vi "CRYInsert Waveform.vi"(8 "sOptionUpdate":string, 9 "sOption":string, 10 "Index":i32[](array[numeric]), 11 "Waveform":T1 {"Y dB ref" format="%.1f"; "Y axis" items=["Log", "Lin"]; "Y data" items=["dB", "Lin"]; "X data" items=["dB", "Lin"]}) -> (2 "Inserted Index":i32[](array[numeric]), 3 "Inserted Name Out":string[](array[string]))   [LabVIEW 2013]
uses:
  CRYSystem/Typedef Control/CRYWaveform Cluster Array.ctl
  CRYSystem/Typedef Control/CRYWaveform Cluster.ctl
  Global/CRYCurve Library Global.vi
  CRYSystem/Task Sequence/CRYProject Run Control Global.vi
  Global/CRYCurves Array Global.vi
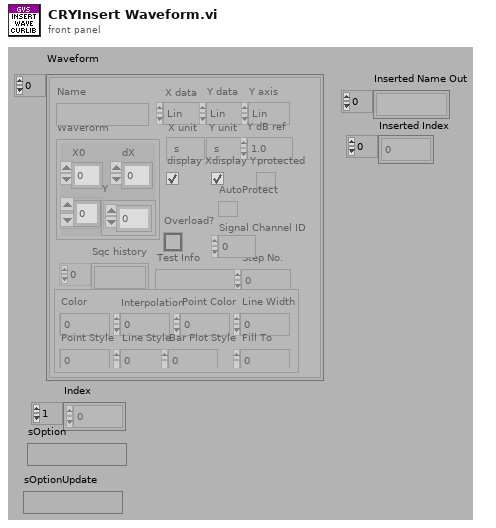
[diagram p1: front panel]
types:
  T1 = typedef "CRYWaveform Cluster Array.ctl" = T2[]
  T2 = typedef "CRYWaveform Cluster.ctl" = cluster{"Waveform":cluster{"X0":dbl, "dX":dbl, "Y":sgl[]}, "X data":u16, "Y data":u16, "Y axis":u16, "X unit":string, "Y unit":string, "Y dB ref":dbl, "display Y":bool, "display X":bool, "Overload?":bool, "Test Info":string, "Step No.":i32, "Name":string, "protected":bool, "Sqc history":string[], "Signal Channel ID":i32, "Plot Settings":cluster{"Color":u32, "Interpolation":u8, "Point Style":u8, "Line Style":u8, "Point Color":u32, "Line Width":u8, "Bar Plot Style":u8, "Fill To":i16}, "AutoProtect":bool}
  T3 = cluster{"Color":u32, "Interpolation":u8, "Point Style":u8, "Line Style":u8, "Point Color":u32, "Line Width":u8, "Bar Plot Style":u8, "Fill To":i16}
  T4 = cluster{"CurveOld":string[], "ValueOld":string[], "ResultOld":string[], "WFMOld":string[], "CurveNew":string[], "ValueNew":string[], "ResultNew":string[], "WFMNew":string[]}
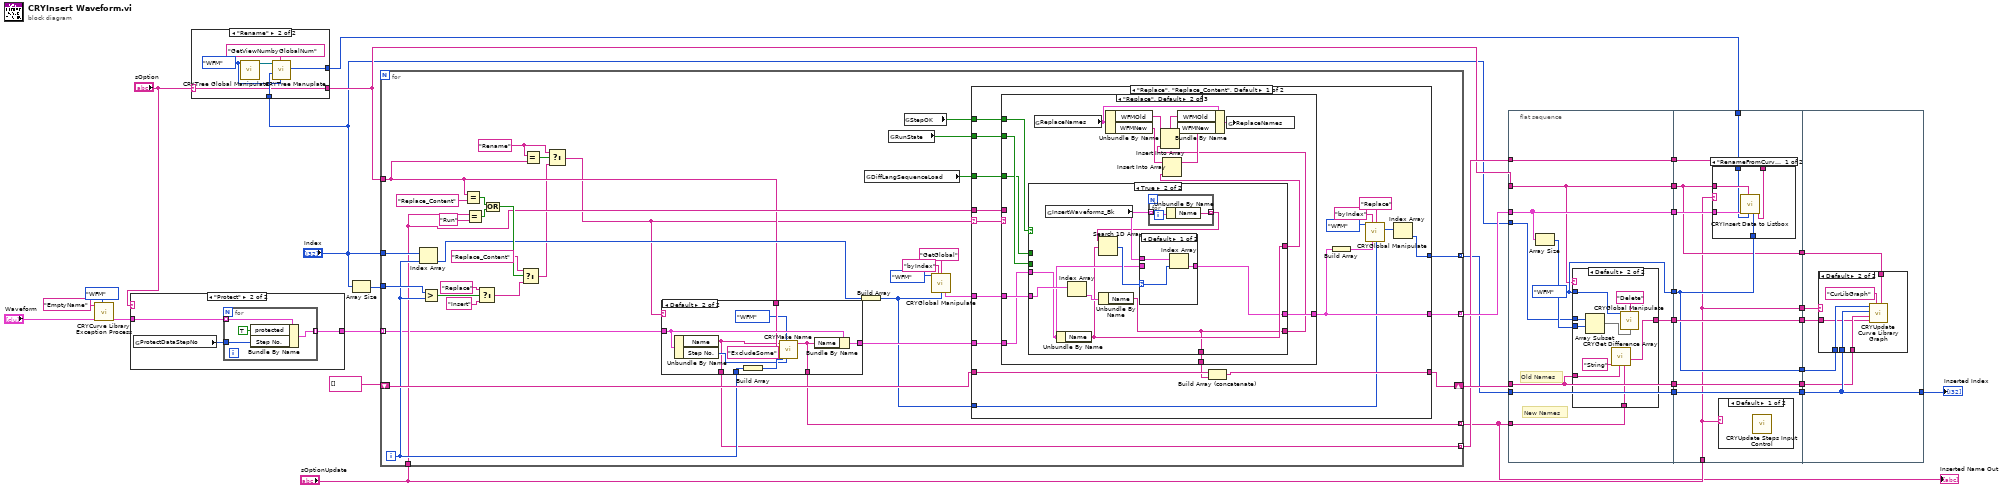
[diagram p0: block diagram]
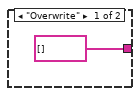
[diagram p4: hidden frame]
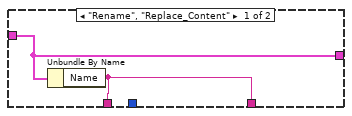
[diagram p8: hidden frame]
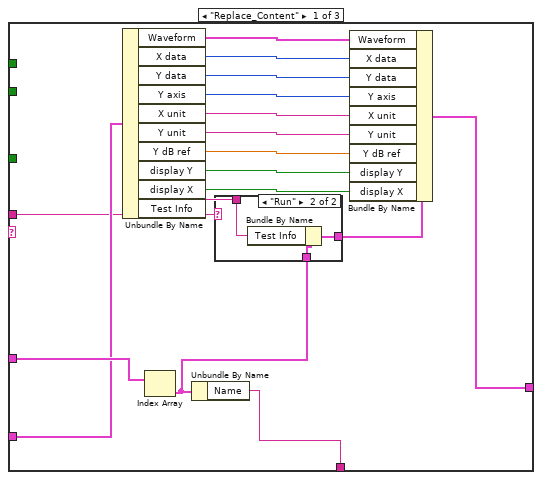
[diagram p9: hidden frame]
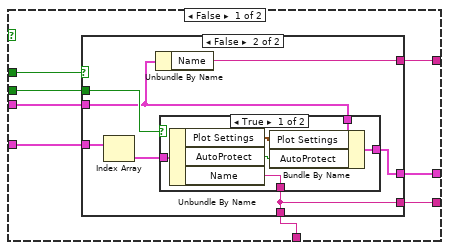
[diagram p11: hidden frame]
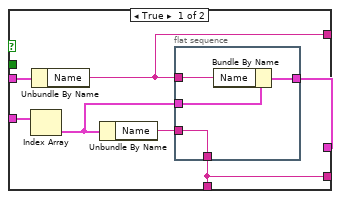
[diagram p12: hidden frame]
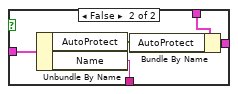
[diagram p13: hidden frame]
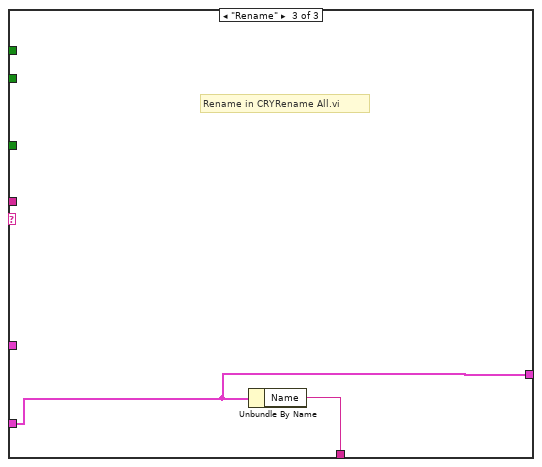
[diagram p15: hidden frame]
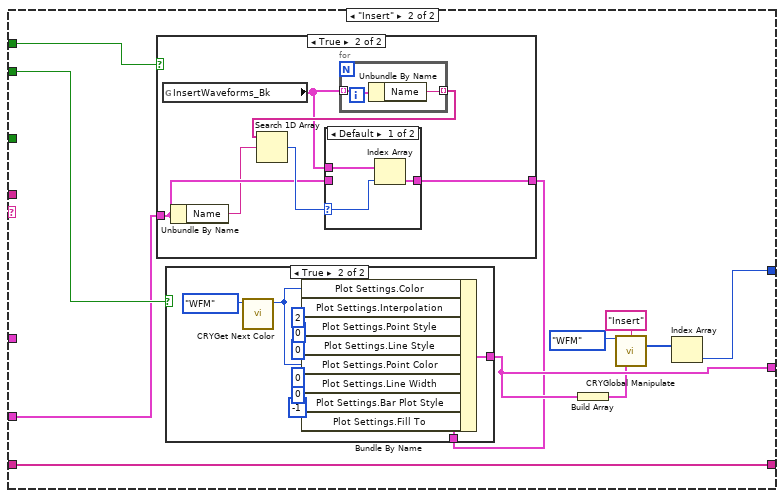
[diagram p16: hidden frame]
diagram:
  n1 = call "CRYCurve Library Exception Process.vi"("Type In"=enum16{"Curves", "Values", "Results", "WFM"}."WFM", "Waveform"="Waveform", "sAction"="EmptyName") -> ("Waveform Out"=w1:T1)  [unwired: 6 in, 2 out]
  n2 = case shown="\"Protect\"" "sOption" {
    tunnel: w1 -> [w32 w35]
    tunnel: [w32 w34] -> w6
    frame Default {
    }
    frame "Protect" {
      n3 = global read "CRYCurve Library Global.vi" "ProtectDataStepNo"() -> (w33:i32)
      n4 = for {
        tunnel: w35 -> [w39] mode=indexing
        tunnel: [w38] -> w34 mode=indexing
        tunnel: w33 -> [w36]
        n5 = Bundle By Name(cluster=w39, "protected"=TRUE, "Step No."=w36) -> (w38:T2)
      }
    }
  }
  n6 = case shown="\"Rename\"" "sOption" {
    selector: "sOption" -> [w40 w42]
    tunnel: "Index" -> [_ w43]
    tunnel: [_ w44] -> w8
    tunnel: [w40 w42] -> w10
    frame Default {
    }
    frame "Rename" {
      w41 = enum16{"Curves", "Values", "Results", "WFM"}."WFM" ("Type In")
      n7 = call "CRYTree Global Manipulate.vi"("Type In"=w41) -> ("Tree/Curve Tree"=w45:refnum<vi>)  [unwired: 7 in, 3 out]
      n8 = call "CRYTree Manuplate.vi"("Type"=w41, "sAction"="GetViewNumbyGlobalNum", "nData"=w43, "Tree in"=w45) -> ("nData Out"=w44:i32[])  [unwired: 4 in, 3 out]
    }
  }
  n9 = Array Size(array="Index") -> (size(s)=w19:i32)
  n10 = for {
    tunnel: [w75] -> w11 mode=indexing
    tunnel: "Index" -> [w72]
    tunnel: w6 -> [w62] mode=indexing
    tunnel: w19 -> [w81]
    shift-right: [w79] -> w30
    shift-left: string[] [] -> [w80]
    tunnel: w10 -> [w52]
    tunnel: [w74] -> w18 mode=indexing
    tunnel: "sOptionUpdate" -> [w63]
    tunnel: [w55] -> w13 mode=indexing
    tunnel: [w48] -> w5 mode=indexing
    i -> [w70]
    w54 = "Rename" ("y")
    n11 = Index Array(array=w72, index=w70) -> (element=w60:i32)
    n12 = Greater?(x=w81, y=w70) -> (0:w76:bool)
    n13 = Equal?(x=w52, y="Replace_Content") -> (x = y?=w67:bool)
    n14 = Equal?(x=w63, y="Run") -> (x = y?=w66:bool)
    n15 = Select(t="Replace" ("sOption"), s=w76, f="Insert" ("sOption")) -> (s? t:f=w71:string)
    n16 = Or(x=w67, y=w66) -> (x .or. y?=w65:bool)
    n17 = Select(t="Replace_Content" ("y"), s=w65, f=w71) -> (s? t:f=w51:string)
    n18 = Equal?(x=w54, y=w52) -> (x = y?=w53:bool)
    n19 = Select(t=w54, s=w53, f=w51) -> (s? t:f=w50:string)
    n20 = case shown="Default" w50 {
      tunnel: [w84 w94] -> w82
      tunnel: w62 -> [w84 w93]
      tunnel: [w83 w92] -> w75
      tunnel: w52 -> [_ w91]
      tunnel: w70 -> [_ w86]
      tunnel: [w83 w85] -> w55
      frame "Rename", "Replace_Content" {
        n21 = Unbundle By Name(w84) -> ("Name"=w83:string)
      }
      frame Default {
        n22 = Unbundle By Name(w93) -> ("Name"=w85:string, "Step No."=w87:i32)
        n23 = Build Array(w86) -> (w88:i32[])
        n24 = call "CRYMake Name.vi"("Step No."=w87, "Type"=enum16{"Curves", "Values", "Results", "WFM"}."WFM", "nData"=w88, "sOption"="ExcludeSome", "sAction"=w91, "Name In"=w85) -> ("Name Out"=w92:string)  [unwired: 4 in, 1 out]
        n25 = Bundle By Name(cluster=w93, "Name"=w92) -> (w94:T2)
      }
    }
    n26 = Build Array(w60) -> (w57:i32[])
    n27 = global read "CRYCurve Library Global.vi" "DiffLangSequenceLoad"() -> (w49:bool)
    n28 = global read "CRYProject Run Control Global.vi" "RunState"() -> (w73:bool)
    n29 = global read "CRYCurve Library Global.vi" "StepOK"() -> (w47:bool)
    n30 = call "CRYGlobal Manipulate.vi"("Type"=enum16{"Curves", "Values", "Results", "WFM"}."WFM", "sOption"="byIndex", "sAction"="GetGlobal", "nData"=w57) -> ("WFM Out"=w61:T2[])  [unwired: 5 in, 6 out]
    n31 = case shown="\"Replace\", \"Replace_Content\", Default" w50 {
      selector: w50 -> [w106 _]
      tunnel: w61 -> [w111 _]
      tunnel: w82 -> [w112 w205]
      tunnel: [w110 w203] -> w79
      tunnel: w80 -> [w109 w203]
      tunnel: [w102 w210] -> w74
      tunnel: w73 -> [w107 w213]
      tunnel: w63 -> [w105 _]
      tunnel: w57 -> [w100 _]
      tunnel: w49 -> [w98 _]
      tunnel: [w96 w207] -> w48
      tunnel: w47 -> [w95 w204]
      frame "Replace", "Replace_Content", Default {
        n32 = case shown="\"Replace\", Default" w106 {
          tunnel: w112 -> [w121 w146 w201]
          tunnel: w111 -> [w122 w148 _]
          tunnel: [w120 w147 w202] -> w108
          tunnel: [w119 w145 w201] -> w102
          tunnel: w107 -> [_ w144 _]
          tunnel: w105 -> [w116 _ _]
          tunnel: w98 -> [_ w143 _]
          tunnel: w95 -> [_ w134 _]
          frame "Replace_Content" {
            n33 = Unbundle By Name(w121) -> ("Waveform"=w123:cluster{"X0":dbl, "dX":dbl, "Y":sgl[]}, "X data"=w124:u16, "Y data"=w125:u16, "Y axis"=w126:u16, "X unit"=w127:string, "Y unit"=w128:string, "Y dB ref"=w129:dbl, "display Y"=w118:bool, "display X"=w117:bool, "Test Info"=w115:string)
            n34 = Index Array(array=w122) -> (element=w114:T2)  [unwired: 1 in]
            n35 = Unbundle By Name(w114) -> ("Name"=w120:string)
            n36 = case shown="\"Run\"" w116 {
              tunnel: w114 -> [w130 w133]
              tunnel: [w130 w132] -> w113
              tunnel: w115 -> [_ w131]
              frame Default {
              }
              frame "Run" {
                n37 = Bundle By Name(cluster=w133, "Test Info"=w131) -> (w132:T2)
              }
            }
            n38 = Bundle By Name(cluster=w113, "Waveform"=w123, "X data"=w124, "Y data"=w125, "Y axis"=w126, "X unit"=w127, "Y unit"=w128, "Y dB ref"=w129, "display Y"=w118, "display X"=w117) -> (w119:T2)
          }
          frame "Replace", Default {
            n39 = case shown="True" w134 {
              tunnel: w148 -> [w156 w190]
              tunnel: [w155 w187] -> w147
              tunnel: w146 -> [w154 w189]
              tunnel: [w153 w186] -> w145
              tunnel: w144 -> [w152 _]
              tunnel: w143 -> [w151 _]
              tunnel: [w150 w188] -> w136
              tunnel: [w149 w187] -> w135
              frame False {
                n40 = case shown="False" w151 {
                  tunnel: w156 -> [w163 w173]
                  tunnel: [w157 w170] -> w155
                  tunnel: w154 -> [w161 w169]
                  tunnel: [w162 w172] -> w153
                  tunnel: w152 -> [_ w171]
                  tunnel: [w158 w168] -> w150
                  tunnel: [w157 w170] -> w149
                  frame True {
                    n41 = Index Array(array=w163) -> (element=w160:T2)  [unwired: 1 in]
                    n42 = Unbundle By Name(w161) -> ("Name"=w158:string)
                    n43 = Unbundle By Name(w160) -> ("Name"=w159:string)
                    n44 = flat-sequence {
                      tunnel: [w167] -> w162
                      tunnel: w160 -> [w166]
                      tunnel: w158 -> [w165]
                      tunnel: w159 -> [w164]
                      tunnel: [w164] -> w157
                      frame #0 {
                        n45 = Bundle By Name(cluster=w166, "Name"=w165) -> (w167:T2)
                      }
                    }
                  }
                  frame False {
                    n46 = Index Array(array=w173) -> (element=w174:T2)  [unwired: 1 in]
                    n47 = Unbundle By Name(w169) -> ("Name"=w168:string)
                    n48 = case shown="True" w171 {
                      tunnel: w174 -> [w180 w185]
                      tunnel: [w179 w184] -> w170
                      tunnel: w169 -> [w178 w183]
                      tunnel: [w176 w181] -> w172
                      frame True {
                        n49 = Unbundle By Name(w180) -> ("Plot Settings"=w175:T3, "AutoProtect"=w177:bool, "Name"=w179:string)
                        n50 = Bundle By Name(cluster=w178, "Plot Settings"=w175, "AutoProtect"=w177) -> (w176:T2)
                      }
                      frame False {
                        n51 = Unbundle By Name(w185) -> ("AutoProtect"=w182:bool, "Name"=w184:string)
                        n52 = Bundle By Name(cluster=w183, "AutoProtect"=w182) -> (w181:T2)
                      }
                    }
                  }
                }
              }
              frame True {
                n53 = global read "CRYCurves Array Global.vi" "InsertWaveforms_Bk"() -> (w193:T1)
                n54 = Unbundle By Name(w189) -> ("Name"=w188:string)
                n55 = Index Array(array=w190) -> (element=w194:T2)  [unwired: 1 in]
                n56 = Unbundle By Name(w194) -> ("Name"=w187:string)
                n57 = for {
                  tunnel: w193 -> [w200] mode=indexing
                  tunnel: [w199] -> w191 mode=indexing
                  n58 = Unbundle By Name(w200) -> ("Name"=w199:string)
                }
                n59 = Search 1D Array(1D array=w191, element=w188) -> (index of element=w192:i32)  [unwired: 1 in]
                n60 = case shown="Default" w192 {
                  selector: w192 -> [w196 _]
                  tunnel: w193 -> [w197 _]
                  tunnel: [w195 w198] -> w186
                  tunnel: w189 -> [_ w198]
                  frame Default {
                    n61 = Index Array(array=w197, index=w196) -> (element=w195:T2)
                  }
                  frame -1 {
                  }
                }
              }
            }
            n62 = global read "CRYCurve Library Global.vi" "ReplaceNames"() -> (w142:T4)
            n63 = Unbundle By Name(w142) -> ("WFMOld"=w140:string[], "WFMNew"=w139:string[])
            n64 = Insert Into Array(array=w140, new element=w135) -> (w138:string[])  [unwired: 1 in]
            n65 = Insert Into Array(array=w139, new element=w136) -> (w137:string[])  [unwired: 1 in]
            n66 = Bundle By Name(cluster=w142, "WFMOld"=w138, "WFMNew"=w137) -> (w141:T4)
            n67 = global write "CRYCurve Library Global.vi" "ReplaceNames"(w141) -> ()
          }
          frame "Rename" {
            # "Rename in CRYRename All.vi"
            n68 = Unbundle By Name(w201) -> ("Name"=w202:string)
          }
        }
        n69 = Build Array (concatenate)(w109, w108) -> (w110:string[])
        n70 = Build Array(w102) -> (w101:T2[])
        n71 = call "CRYGlobal Manipulate.vi"("Type"=enum16{"Curves", "Values", "Results", "WFM"}."WFM", "sOption"="byIndex", "sAction"="Replace", "WFM"=w101, "nData"=w100) -> ("nData out"=w97:i32[])  [unwired: 4 in, 6 out]
        n72 = Index Array(array=w97) -> (element=w96:i32)  [unwired: 1 in]
      }
      frame "Insert" {
        n73 = case shown="True" w204 {
          tunnel: w205 -> [w214 w217]
          tunnel: [w214 w216] -> w206
          frame False {
          }
          frame True {
            n74 = global read "CRYCurves Array Global.vi" "InsertWaveforms_Bk"() -> (w218:T1)
            n75 = Unbundle By Name(w217) -> ("Name"=w215:string)
            n76 = for {
              tunnel: w218 -> [w226] mode=indexing
              tunnel: [w225] -> w220 mode=indexing
              n77 = Unbundle By Name(w226) -> ("Name"=w225:string)
            }
            n78 = Search 1D Array(1D array=w220, element=w215) -> (index of element=w219:i32)  [unwired: 1 in]
            n79 = case shown="Default" w219 {
              selector: w219 -> [w222 _]
              tunnel: w218 -> [w223 _]
              tunnel: [w221 w224] -> w216
              tunnel: w217 -> [_ w224]
              frame Default {
                n80 = Index Array(array=w223, index=w222) -> (element=w221:T2)
              }
              frame -1 {
              }
            }
          }
        }
        n81 = case shown="True" w213 {
          tunnel: w206 -> [w227 w230]
          tunnel: [w227 w229] -> w210
          frame False {
          }
          frame True {
            n82 = call "CRYGet Next Color.vi"("Type"=enum16{"Curves", "Values", "Results", "WFM"}."WFM") -> ("Color"=w234:u32)  [unwired: 10 out]
            n83 = Bundle By Name(cluster=w230, "Plot Settings.Color"=w234, "Plot Settings.Interpolation"=u8 2, "Plot Settings.Point Style"=u8 0, "Plot Settings.Line Style"=u8 0, "Plot Settings.Point Color"=w234, "Plot Settings.Line Width"=u8 0, "Plot Settings.Bar Plot Style"=u8 0, "Plot Settings.Fill To"=i16 -1) -> (w229:T2)
          }
        }
        n84 = Build Array(w210) -> (w209:T2[])
        n85 = call "CRYGlobal Manipulate.vi"("Type"=enum16{"Curves", "Values", "Results", "WFM"}."WFM", "sAction"="Insert", "WFM"=w209) -> ("nData out"=w208:i32[])  [unwired: 6 in, 6 out]
        n86 = Index Array(array=w208) -> (element=w207:i32)  [unwired: 1 in]
      }
    }
  }
  "Inserted Name Out" <- w11
  n87 = flat-sequence {
    tunnel: [w247] -> w31
    tunnel: w18 -> [w247]
    tunnel: "Index" -> [w244]
    tunnel: w30 -> [w239]
    tunnel: w11 -> [w238]
    tunnel: [w246] -> w29
    tunnel: [w239] -> w28
    tunnel: [w243] -> w25
    tunnel: w5 -> [w242]
    tunnel: [w242] -> w22
    tunnel: [w241] -> w20
    tunnel: w10 -> [w241]
    tunnel: w13 -> [w240]
    tunnel: [w240] -> w12
    tunnel: [w266] -> w27
    tunnel: [w265] -> w26
    tunnel: w28 -> [w265]
    tunnel: w29 -> [w266]
    tunnel: w31 -> [w264]
    tunnel: w25 -> [w262]
    tunnel: [w262] -> w24
    tunnel: [w263] -> w23
    tunnel: w22 -> [w263]
    tunnel: w20 -> [w260]
    tunnel: [w260] -> w16
    tunnel: "sOptionUpdate" -> [w258]
    tunnel: [w258] -> w15
    tunnel: w12 -> [w261]
    tunnel: w8 -> [w259]
    tunnel: w27 -> [w274]
    tunnel: w26 -> [w275]
    tunnel: w24 -> [w277]
    tunnel: w23 -> [w276]
    tunnel: [w276] -> w17
    tunnel: w16 -> [w273]
    tunnel: w15 -> [w272]
    frame #0 {
      w243 = enum16{"Curves", "Values", "Results", "WFM"}."WFM" ("Type")
      # "New Names"
      # "Old Names"
      n88 = Array Size(array=w247) -> (size(s)=w245:i32)
      n89 = case shown="Default" w241 {
        tunnel: [string[] [] ("Deleted Names") w249] -> w246
        tunnel: w245 -> [_ w257]
        tunnel: w244 -> [_ w256]
        tunnel: w243 -> [_ w253]
        tunnel: w239 -> [_ w251]
        tunnel: w238 -> [_ w250]
        frame "Overwrite" {
        }
        frame Default {
          n90 = Array Subset(array=w256, index=w257) -> (w254:i32[])  [unwired: 1 in]
          n91 = call "CRYGet Difference Array.vi"("String2"=w250, "String1"=w251, "sOption"="String") -> ("StringDiff Out"=w249:string[])  [unwired: 7 in, 1 out]
          n92 = call "CRYGlobal Manipulate.vi"("Type"=w253, "sAction"="Delete", "nData"=w254) -> ()  [unwired: 6 in, 7 out]
        }
      }
    }
    frame #1 {
      n93 = case shown="\"RenameFromCurve\", Default" w258 {
        tunnel: w264 -> [w270 _]
        tunnel: w262 -> [w271 _]
        tunnel: w261 -> [w269 _]
        tunnel: w260 -> [w268 _]
        tunnel: w259 -> [w267 _]
        frame "RenameFromCurve", Default {
          n94 = call "CRYInsert Data to Listbox.vi"("OrgNames"=w269, "Type"=w271, "nData"=w267, "sOption"=w268, "Waveforms"=w270) -> ()  [unwired: 6 in, 1 out]
        }
        frame "Run" {
        }
      }
      n95 = case shown="Default" w258 {
        frame Default {
          n96 = call "CRYUpdate Steps Input Control.vi"() -> ()  [unwired: 12 in]
        }
        frame "AddStep", "Apply", "Run" {
        }
      }
    }
    frame #2 {
      n97 = case shown="Default" w272 {
        tunnel: w277 -> [_ w282]
        tunnel: w276 -> [_ w281]
        tunnel: w275 -> [_ w280]
        tunnel: w274 -> [_ w279]
        tunnel: w273 -> [_ w278]
        frame "RenameFromCurve", "Run" {
        }
        frame Default {
          n98 = call "CRYUpdate Curve Library Graph.vi"("sOption 2"=w278, "sOption 1"="CurLibGraph" ("sOption"), "Deleted Names"=w279, "Replaced Old Names"=w280, "Index"=w281, "Type"=w282) -> ()  [unwired: 6 in]
        }
      }
    }
  }
  "Inserted Index" <- w17
